vi "Parse Results Array (single).vi"(6 "Datatype":T1, 7 "Processing":enum16{"Mean", "Sample"}(ring), 8 "error in (no error)":errorcluster, 9 "Reference Channel":i32=1, 10 "AI Channel":i32=1, 11 "Results (Dictionary)":cluster{"key":string, "value":dbl[]}[](array[cluster])) -> (0 "error out":errorcluster, 1 "Name":string, 2 "Data":dbl, 3 "Results (Dictionary)":cluster{"key":string, "value":dbl[]}[](array[cluster]))   [LabVIEW 2019, in "Instrument.Lockin.lvlib" / "Instrument.Lockin.lvclass"]
doc: "This method will search the <b>Results Dictionary</b> for the data specified by <b>Datatype</b>, <b>AI Channel</b>, and <b>Ref Channel</b>.\n\n<b>Data</b> is either samples one point or takes the mean of the returned array values in the matched channel."
uses:
  Instrument.Lockin.lvclass
  <vilib>/Analysis/NI_AALBase.lvlib
  <vilib>/Analysis/baseanly.llb/Mean (DBL).vi
  Typedefs/Results Type--Enum.ctl
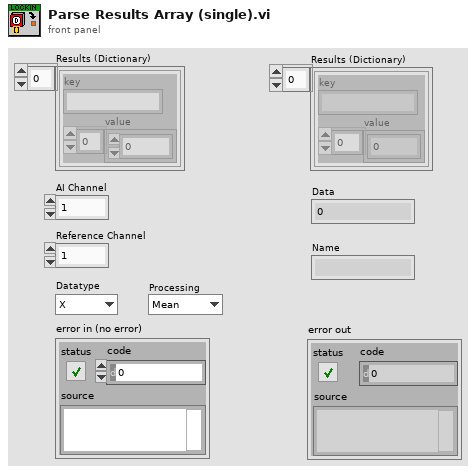
[diagram p1: front panel]
types:
  T1 = typedef "Instrument.Lockin.lvlib/Instrument.Lockin.lvclass/Results Type--Enum.ctl" = enum16{"X", "Y", "R", "Theta", "Mean"}
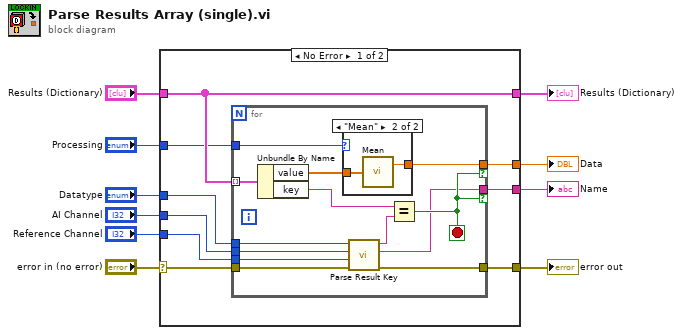
[diagram p0: block diagram]
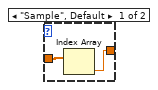
[diagram p2: hidden frame]
diagram:
  n1 = case shown="No Error" "error in (no error)" {
    selector: "error in (no error)" -> [w15 w37]
    tunnel: "Datatype" -> [w18 _]
    tunnel: "Results (Dictionary)" -> [w19 w38]
    tunnel: [w16 _] -> w4
    tunnel: [w14 w37] -> w3
    tunnel: [w19 w38] -> w7
    tunnel: "Reference Channel" -> [w17 _]
    tunnel: "AI Channel" -> [w12 _]
    tunnel: [w13 _] -> w2
    tunnel: "Processing" -> [w11 _]
    frame No Error {
      n2 = for {
        tunnel: [w24] -> w13 if=w28
        tunnel: [w27] -> w16 if=w28
        tunnel: w19 -> [w31] mode=indexing
        tunnel: w12 -> [w21]
        tunnel: w17 -> [w20]
        tunnel: w18 -> [w30]
        tunnel: w15 -> [w26]
        tunnel: [w25] -> w14
        tunnel: w11 -> [w22]
        stop <- w28 stop-if-true
        n3 = Unbundle By Name(w31) -> ("value"=w32:dbl[], "key"=w23:string)
        n4 = case shown="\"Mean\"" w22 {
          tunnel: w32 -> [w34 w36]
          tunnel: [w33 w35] -> w24
          frame "Sample", Default {
            n5 = Index Array(array=w34) -> (element=w33:dbl)  [unwired: 1 in]
          }
          frame "Mean" {
            n6 = call-poly <vilib>:"Mean.vi"("X"=w36) -> ("mean"=w35:dbl)  [unwired: 1 out]
          }
        }
        n7 = call "Parse Result Key.vi"("error in (no error)"=w26, "Ref Channel"=w20, "AI Channel"=w21, "Datatype"=w30) -> ("error out"=w25:errorcluster, "Label"=w27:string, "Key"=w29:string)  [unwired: 5 in]
        n8 = Equal?(x=w23, y=w29) -> (x = y?=w28:bool)
      }
    }
    frame Error {
    }
  }
  "Data" <- w2
  "Results (Dictionary)" <- w7
  "Name" <- w4
  "error out" <- w3
